vi "Chroma 1905x Series Ramp Time Results.vi"(0 "inst handle Out":refnum<visa-resource-name>, 1 "error in":T1) -> (2 "inst handle in":refnum<visa-resource-name>, 3 "Result":string, 5 "error out":T1)   [LabVIEW 2025]
uses:
  <instrlib>/Chroma 19052/Chroma 19052.lvlib
panel:
  # "Ramp Time Results"
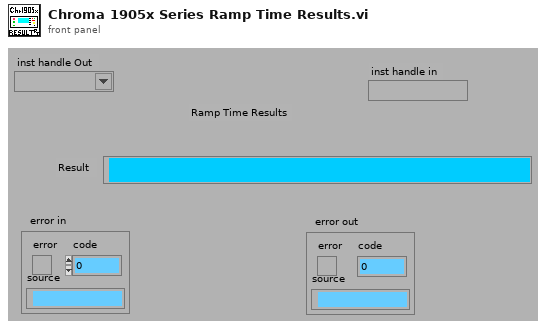
[diagram p1: front panel]
types:
  T1 = cluster{"error":bool, "code":i8, "source":string}
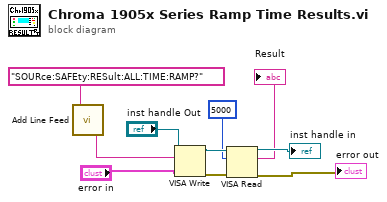
[diagram p0: block diagram]
diagram:
  n1 = call <instrlib>:"Add Line Feed.vi"("Cmdstring"="SOURce:SAFEty:RESult:ALL:TIME:RAMP?") -> ("Concatenated String"=w1:string)
  n2 = VISA Write(VISA resource name="inst handle Out", write buffer=w1, error in (no error)="error in") -> (VISA resource name out=w8:refnum<visa-resource-name>, error out=w7:errorcluster)  [unwired: 1 out]
  n3 = VISA Read(VISA resource name=w8, byte count=5000, error in (no error)=w7) -> (VISA resource name out=→"inst handle in":refnum<visa-resource-name>, read buffer=→"Result":string, error out=→"error out":errorcluster)  [unwired: 1 out]
